vi "Vorschau Stoermeldungen.vi"() -> (0 "Vorschau Störungen":string[](array[string]), 2 "Störungsnummern":i32[](array[numeric]))   [LabVIEW 2020, in "Stoerungen.lvlib"]
uses:
  Stoerungen.lvlib
  FGV Stoerungsdatei Aktionen.ctl
  FGV Stoermeldungen Aktion.ctl
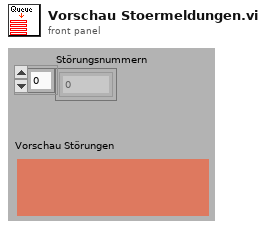
[diagram p1: front panel]
types:
  T1 = typedef "Stoerungen.lvlib/FGV Stoermeldungen Aktion.ctl" = enum16{"Initialisieren", "kommend", "gehend", "lesen", "Queue leeren", "Queue freigeben", "in Datei loggen", "Änderung zurücksetzen"}
  T2 = typedef "Stoerungen.lvlib/FGV Stoerungsdatei Aktionen.ctl" = enum16{"lesen", "laden", "Neue Werte"}
  T3 = typedef "Stoerungen.lvlib/Stoermeldung.ctl" = cluster{"Zeitstempel":timestamp, "Nummer":i32, "Kommend":bool}
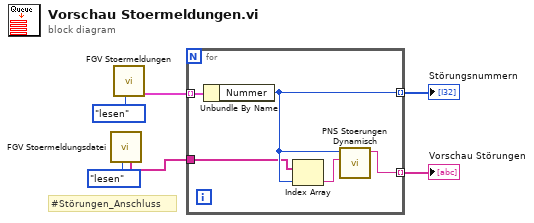
[diagram p0: block diagram]
diagram:
  # "#Störungen_Anschluss"
  n1 = call "FGV Stoermeldungsdatei.vi"("Aktionen"=FGV_Stoerungsdatei_Aktionen."lesen") -> ("Text"=w1:string[])  [unwired: 2 in, 8 out]
  n2 = call "FGV Stoermeldungen.vi"("Aktion"=FGV_Stoermeldungen_Aktion."lesen") -> ("Anzeige Array"=w2:T3[])  [unwired: 3 in, 7 out]
  n3 = for {
    tunnel: w1 -> [w8]
    tunnel: w2 -> [w11] mode=indexing
    tunnel: [w9] -> w6 mode=indexing
    tunnel: [w10] -> w4 mode=indexing
    n4 = Unbundle By Name(w11) -> ("Nummer"=w9:i32)
    n5 = Index Array(array=w8, index=w9) -> (element=w7:string)
    n6 = call "PNS Stoerungen Dynamisch.vi"("Störmeldetexte"=w7, "Nummer"=w9) -> ("String"=w10:string)  [unwired: 9 in]
  }
  "Störungsnummern" <- w6
  "Vorschau Störungen" <- w4
